vi "Write Status.vi"(8 "error in (no error)":errorcluster, 10 "Status":T1, 11 "PD-Data in":refnum<class "HC-Main.lvclass">) -> (0 "error out":errorcluster, 3 "PD-Data out":refnum<class "HC-Main.lvclass">)   [LabVIEW 2013, in "HardwareCharacterization.lvlib" / "HC-Main.lvclass"]
uses:
  HC-Main.lvclass
  Application-status.ctl
  HC-Main.lvclass/HC-Main.ctl
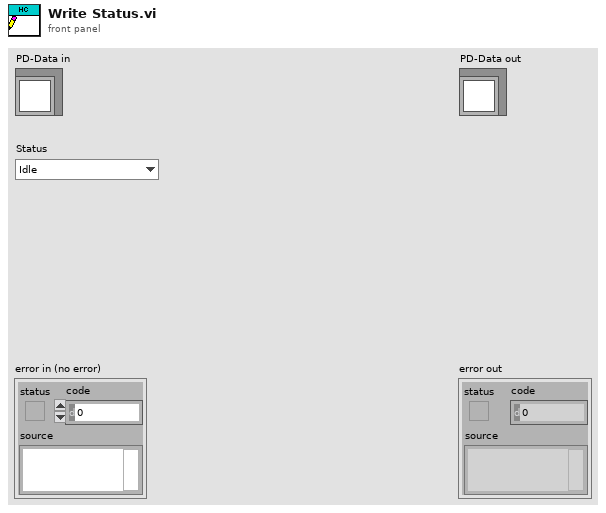
[diagram p1: front panel]
types:
  T1 = typedef "HardwareCharacterization.lvlib/HC-Main.lvclass/Application-status.ctl" = enum16{"Idle", "Initialized", "Configured", "Activated", "Started", "Paused", "Stopped", "Reset", "Error", "Exited"}
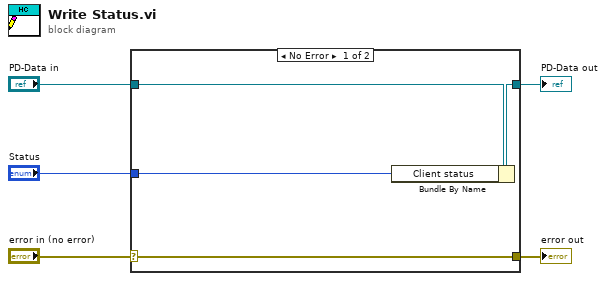
[diagram p0: block diagram]
diagram:
  n1 = case shown="No Error" "error in (no error)" {
    selector: "error in (no error)" -> [w9 w10]
    tunnel: [w9 w10] -> w4
    tunnel: [w7 w11] -> w2
    tunnel: "PD-Data in" -> [w8 w11]
    tunnel: "Status" -> [w6 _]
    frame No Error {
      n2 = Bundle By Name(cluster=w8, "Client status"=w6) -> (w7:refnum<class "HC-Main.lvclass">)
    }
    frame Error {
    }
  }
  "error out" <- w4
  "PD-Data out" <- w2
